vi "Run Virtual Key Entries.vi"(8 "error in (no error)":errorcluster, 11 "Key Press Array":u8[][](array[numeric])) -> (0 "error out":errorcluster)   [LabVIEW 2020, in "MacroAssert.lvlib" / "Win Util.lvlib"]
uses:
  Win Util.lvlib
  user32.dll
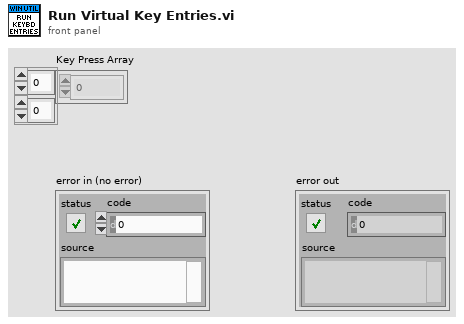
[diagram p1: front panel]
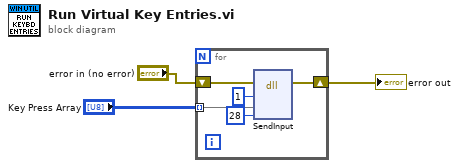
[diagram p0: block diagram]
diagram:
  n1 = for {
    tunnel: "Key Press Array" -> [w8] mode=indexing
    shift-right: [w4] -> w1
    shift-left: "error in (no error)" -> [w5]
    n2 = dll-call lib="user32.dll" fn="SendInput"(error in=w5, "nInputs"=u32 1, "pInputs"=w8, "cbSize"=28) -> (error out=w4:errorcluster)  [unwired: 6 in, 1 out]
  }
  "error out" <- w1
